vi "get index definition.vi"(10 "channel classification":T1, 11 "Custom Controller Module configuration in":refnum<class "Custom Controller Module configuration.lvclass">) -> (1 "valid?":bool, 2 "index cluster":variant, 3 "Custom Controller Module configuration out":refnum<class "Custom Controller Module configuration.lvclass">)   [LabVIEW 2013, in "Custom Controller Module configuration.lvclass"]
uses:
  Custom Controller Module configuration.lvclass
  <vilib>/NI/Tag Bus Module Framework/channel/channel classification.ctl
  input data indices.ctl
  output data indices.ctl
  parameter data indices.ctl
  result data indices.ctl
  <vilib>/NI/Tag Bus Module Framework/channel/TBM channel.lvclass
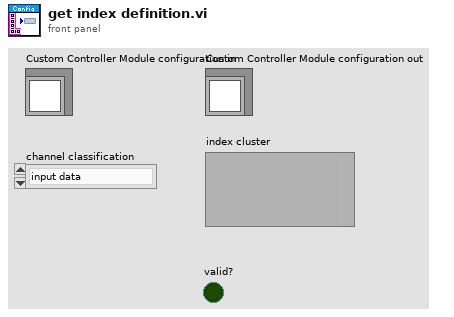
[diagram p1: front panel]
types:
  T1 = typedef "TBM channel.lvclass/channel classification.ctl" = enum16{"input data", "output data", "processing parameter", "processing result"}
  T2 = typedef "Custom Controller Module configuration.lvclass/input data indices.ctl" = cluster{"fmwk_placeholder":i32}
  T3 = typedef "Custom Controller Module configuration.lvclass/output data indices.ctl" = cluster{"fmwk_placeholder":i32}
  T4 = typedef "Custom Controller Module configuration.lvclass/parameter data indices.ctl" = cluster{"Double.Temperature":i32, "Double.setpoint":i32, "Double.output range high":i32, "Double.output range low":i32, "Double.Kc":i32, "Double.Ti":i32, "Double.Td":i32, "Boolean.Fan on?":i32}
  T5 = typedef "Custom Controller Module configuration.lvclass/result data indices.ctl" = cluster{"Double.fan":i32, "Double.lamp":i32}
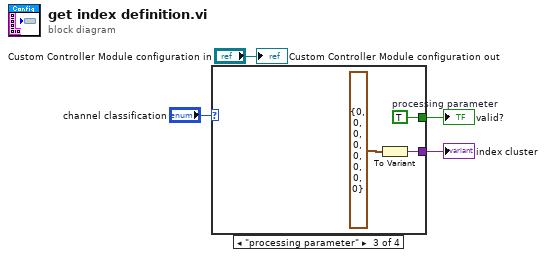
[diagram p0: block diagram]
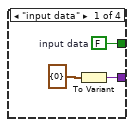
[diagram p2: hidden frame]
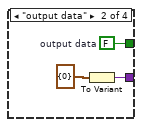
[diagram p3: hidden frame]
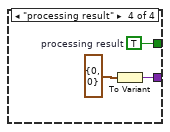
[diagram p4: hidden frame]
diagram:
  n1 = case shown="\"processing parameter\"" "channel classification" {
    tunnel: [w6 w10 w13 w16] -> w2
    tunnel: [w5 w9 w12 w15] -> w1
    frame "input data" {
      w5 = FALSE  # input data
      n2 = To Variant(anything=T2 {"fmwk_placeholder"=0} ("Cluster")) -> (Variant=w6:variant)
    }
    frame "output data" {
      w9 = FALSE  # output data
      n3 = To Variant(anything=T3 {"fmwk_placeholder"=0} ("Cluster")) -> (Variant=w10:variant)
    }
    frame "processing parameter" {
      w12 = TRUE  # processing parameter
      n4 = To Variant(anything=T4 {"Double.Temperature"=0, "Double.setpoint"=0, "Double.output range high"=0, "Double.output range low"=0, "Double.Kc"=0, "Double.Ti"=0, "Double.Td"=0, "Boolean.Fan on?"=0} ("Cluster")) -> (Variant=w13:variant)
    }
    frame "processing result" {
      w15 = TRUE  # processing result
      n5 = To Variant(anything=T5 {"Double.fan"=0, "Double.lamp"=0} ("Cluster")) -> (Variant=w16:variant)
    }
  }
  "index cluster" <- w2
  "valid?" <- w1
  "Custom Controller Module configuration out" <- "Custom Controller Module configuration in"
